vi "perform-autocomplete.vi"(11 "Path in":refnum<vi>) -> ()   [LabVIEW 2020, in "path-with-auto-complete.lvclass"]
uses:
  path-with-auto-complete.lvclass
  <vilib>/Utility/miscctls.llb/LVSelectionTypeDef.ctl
  path-with-auto-complete.lvclass/path-with-auto-complete.ctl
panel:
  out "error out":errorcluster
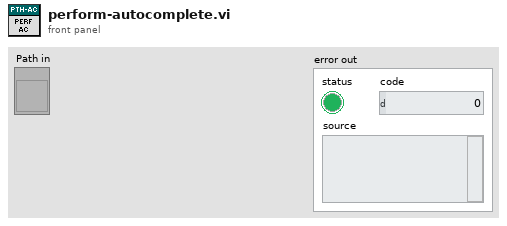
[diagram p1: front panel]
types:
  T1 = typedef "LVSelectionTypeDef.ctl" = cluster{"Selection Start":u32, "Selection End":u32}
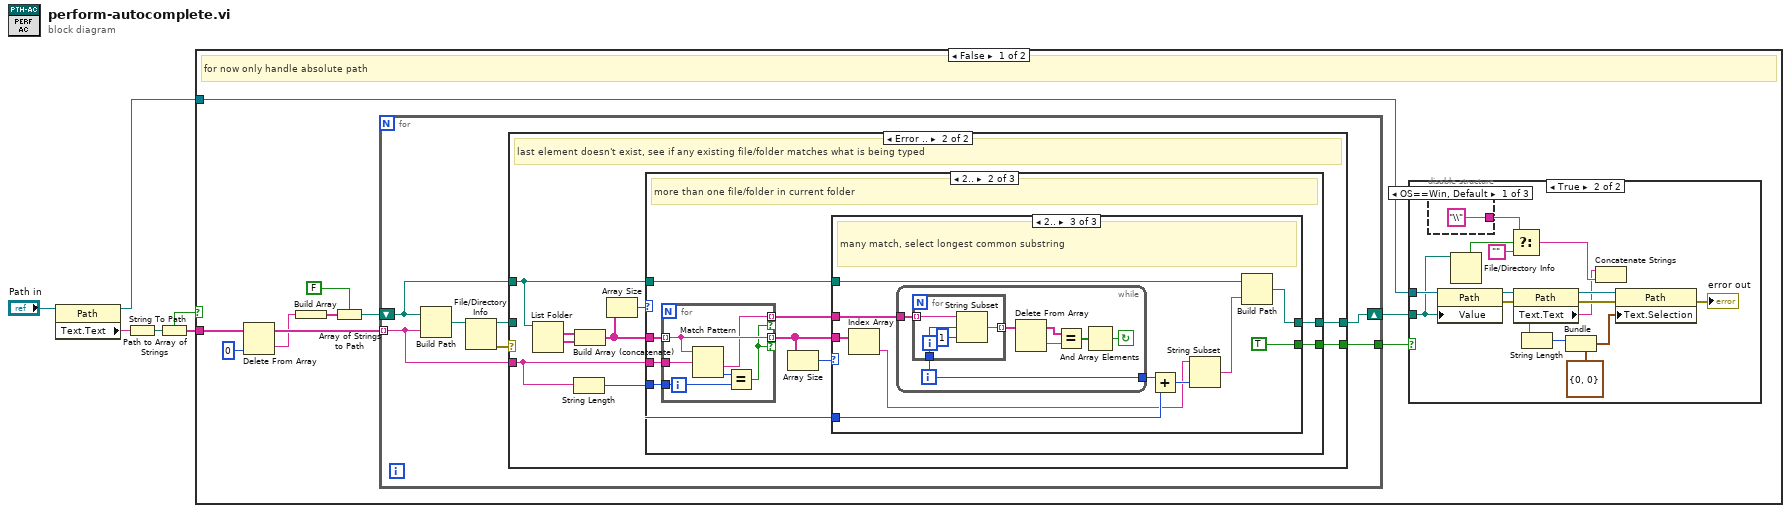
[diagram p0: block diagram]
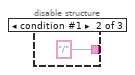
[diagram p3: hidden frame]
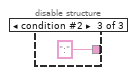
[diagram p4: hidden frame]
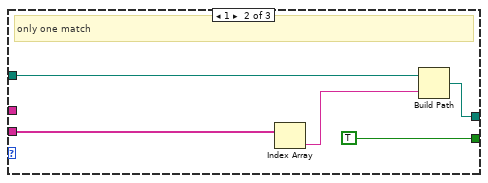
[diagram p8: hidden frame]
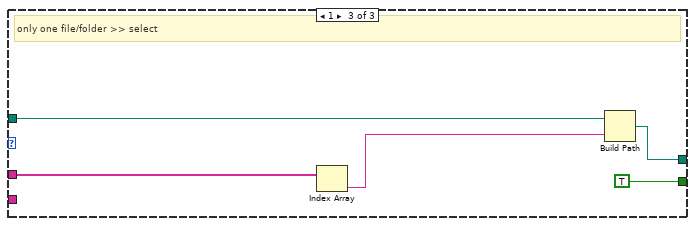
[diagram p9: hidden frame]
diagram:
  n1 = property class="Path"(reference="Path in") -> (reference out=w5:refnum<vi>, "Text.Text"=w4:string)  [unwired: 1 in, 1 out]
  n2 = String To Path(string=w4) -> (path=w3:path)
  n3 = Path to Array of Strings(0:w3) -> (1:w1:bool, 2:w2:string[])
  n4 = case shown="False" w1 {
    tunnel: w2 -> [w16 _]
    tunnel: w5 -> [w7 _]
    frame False {
      # "for now only handle absolute path"
      n5 = Delete From Array(array=w16, index=0) -> (deleted portion=w13:string, array with subset deleted=w15:string[])  [unwired: 1 in]
      n6 = Build Array(w13) -> (w11:string[])
      n7 = Array of Strings to Path(0:w11, 1:FALSE ("relative")) -> (2:w12:path)
      n8 = for {
        shift-right: [w39] -> w8
        shift-left: w12 -> [w37]
        tunnel: w15 -> [w36] mode=indexing
        tunnel: [w35] -> w9
        n9 = Build Path(base path=w37, name or relative path=w36) -> (appended path=w41:path)
        n10 = File/Directory Info(path=w41) -> (path out=w38:path, error out=w40:errorcluster)  [unwired: 1 in, 5 out]
        n11 = case shown="Error .." w40 {
          tunnel: [w42 w47] -> w39
          tunnel: w38 -> [w42 _]
          tunnel: w37 -> [_ w48]
          tunnel: w36 -> [_ w49]
          tunnel: [_ w46] -> w35
          frame No Error {
            # "file or folder exists, nothing to do"
          }
          frame Error {
            # "last element doesn't exist, see if any existing file/folder matches what is being typed"
            n12 = List Folder(path=w48) -> (filenames=w51:string[], folder names=w50:string[])  [unwired: 3 in, 2 out]
            n13 = String Length(string=w49) -> (length=w45:i32)
            n14 = Build Array (concatenate)(w51, w50) -> (w44:string[])
            n15 = Array Size(array=w44) -> (size(s)=w43:i32)
            n16 = case shown="2.." w43 {
              tunnel: w49 -> [_ w61 _]
              tunnel: w48 -> [w52 w58 w98]
              tunnel: [w52 w57 w97] -> w47
              tunnel: [_ w56 TRUE] -> w46
              tunnel: w45 -> [_ w54 _]
              tunnel: w44 -> [_ w53 w95]
              frame ..0 {
                # "empty folder"
              }
              frame 2.. {
                # "more than one file/folder in current folder"
                n17 = for {
                  tunnel: w53 -> [w93] mode=indexing
                  tunnel: w61 -> [w91]
                  tunnel: [w93] -> w59 mode=indexing if=w88
                  tunnel: w54 -> [w90]
                  tunnel: [w89] -> w55 mode=indexing if=w88
                  n18 = Match Pattern(string=w93, regular expression=w91) -> (after substring=w89:string, offset past match=w92:i32)  [unwired: 1 in, 2 out]
                  n19 = Equal?(x=w92, y=w90) -> (x = y?=w88:bool)
                }
                n20 = Array Size(array=w59) -> (size(s)=w60:i32)
                n21 = case shown="2.." w60 {
                  tunnel: w59 -> [_ w65 w68]
                  tunnel: w58 -> [_ w66 w76]
                  tunnel: [_ w63 w75] -> w57
                  tunnel: [_ TRUE TRUE] -> w56
                  tunnel: w55 -> [_ _ w73]
                  tunnel: w54 -> [_ _ w70]
                  frame ..0 {
                    # "no match"
                  }
                  frame 1 {
                    # "only one match"
                    n22 = Index Array(array=w65) -> (element=w64:string)  [unwired: 1 in]
                    n23 = Build Path(base path=w66, name or relative path=w64) -> (appended path=w63:path)
                  }
                  frame 2.. {
                    # "many match, select longest common substring"
                    n24 = Index Array(array=w68) -> (element=w67:string)  [unwired: 1 in]
                    n25 = while {
                      tunnel: [w78] -> w72
                      tunnel: w73 -> [w77]
                      i -> [w78]
                      stop <- w79 continue-if-true
                      n26 = for {
                        tunnel: w77 -> [w87] mode=indexing
                        tunnel: [w85] -> w83 mode=indexing
                        tunnel: w78 -> [w84]
                        n27 = String Subset(string=w87, offset (0)=w84, length (rest)=1 ("length (rest)")) -> (substring=w85:string)
                      }
                      n28 = Delete From Array(array=w83) -> (deleted portion=w82:string, array with subset deleted=w81:string[])  [unwired: 2 in]
                      n29 = Equal?(x=w81, y=w82) -> (x = y?=w80:bool[])
                      n30 = And Array Elements(Boolean array=w80) -> (logical AND=w79:bool)
                    }
                    n31 = Add(x=w72, y=w70) -> (x+y=w71:i32)
                    n32 = String Subset(string=w67, length (rest)=w71) -> (substring=w69:string)  [unwired: 1 in]
                    n33 = Build Path(base path=w76, name or relative path=w69) -> (appended path=w75:path)
                  }
                }
              }
              frame 1 {
                # "only one file/folder >> select"
                n34 = Index Array(array=w95) -> (element=w94:string)  [unwired: 1 in]
                n35 = Build Path(base path=w98, name or relative path=w94) -> (appended path=w97:path)
              }
            }
          }
        }
      }
      n36 = case shown="True" w9 {
        tunnel: w8 -> [_ w30]
        tunnel: w7 -> [_ w31]
        frame False {
        }
        frame True {
          n37 = disable-structure shown="OS==Win, Default" {
            disable-tunnel: ["\\" "/" ":"] -> w26
            frame condition #0 (active) {
            }
            frame condition #1 {
            }
            frame condition #2 {
            }
          }
          n38 = property class="Path"(reference=w31, "Value"=w30) -> (reference out=w21:refnum<vi>, error out=w19:errorcluster)  [unwired: 1 in]
          n39 = File/Directory Info(path=w30) -> (directory=w29:bool)  [unwired: 1 in, 6 out]
          n40 = Select(t=w26, s=w29, f="") -> (s? t:f=w28:string)
          n41 = property class="Path"(reference=w21, error in=w19) -> (reference out=w20:refnum<vi>, error out=w18:errorcluster, "Text.Text"=w17:string)
          n42 = String Length(string=w17) -> (length=w23:i32)
          n43 = Bundle(cluster=T1 {"Selection Start"=0, "Selection End"=0} ("Path Text.Selection"), "Selection Start"=w23) -> (w24:T1)  [unwired: 1 in]
          n44 = Concatenate Strings(w17, w28) -> ()  [unwired: 1 out]
          n45 = property class="Path"(reference=w20, error in=w18, "Text.Selection"=w24) -> (error out=→"error out":errorcluster)  [unwired: 1 out]
        }
      }
    }
    frame True {
      # "i don't know where to start from..."
    }
  }
